vi "Write power_.vi"(8 "error in (no error)":errorcluster, 10 "power?":bool, 11 "Update Meerstetter Ctl Val in":refnum<class "Update Meerstetter Ctl Val.lvclass">) -> (0 "error out":errorcluster, 3 "Update Meerstetter Ctl Val out":refnum<class "Update Meerstetter Ctl Val.lvclass">)   [LabVIEW 2014, in "Controller.lvlib" / "Update Meerstetter Ctl Val.lvclass"]
uses:
  Update Meerstetter Ctl Val.lvclass
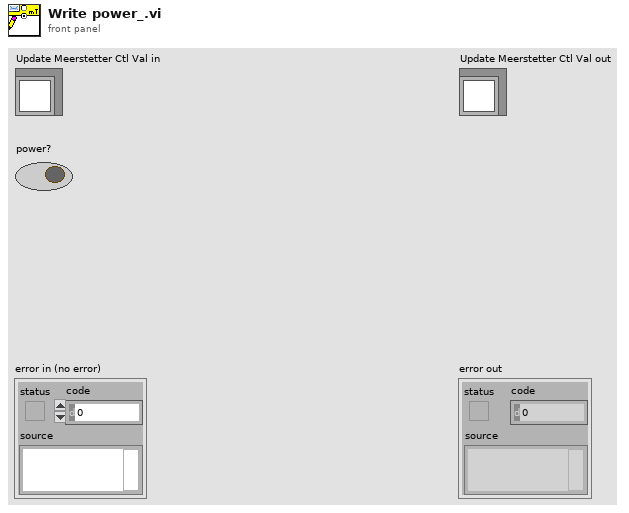
[diagram p1: front panel]
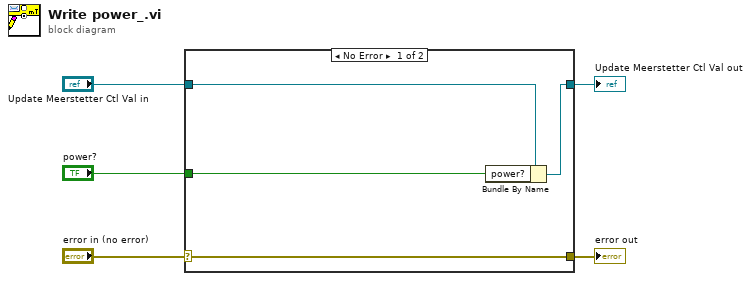
[diagram p0: block diagram]
diagram:
  n1 = case shown="No Error" "error in (no error)" {
    selector: "error in (no error)" -> [w9 w10]
    tunnel: [w9 w10] -> w4
    tunnel: [w7 w11] -> w2
    tunnel: "Update Meerstetter Ctl Val in" -> [w8 w11]
    tunnel: "power?" -> [w6 _]
    frame No Error {
      n2 = Bundle By Name(cluster=w8, "power?"=w6) -> (w7:refnum<class "Update Meerstetter Ctl Val.lvclass">)
    }
    frame Error {
    }
  }
  "error out" <- w4
  "Update Meerstetter Ctl Val out" <- w2
